vi "UIM Resolution.vi"() -> ()   [LabVIEW 2020]
doc: "This example shows how you could use UIM API to modify the resolution and layout of your application. Like this you can easily adapt your UI to different monitors."
uses:
  <vilib>/Utility/miscctls.llb/LVRectTypeDef.ctl
  UIM Class/UIM.lvclass
panel:
  in  "XML File":path caption="UIM XML Path"
  in  "Tab Control":enum32{"Page 1", "Page 2"}(tab)
  in  "Listbox":i32(listbox)
  in  "Play Button":bool
  in  "String":string
  out "Waveform Graph":dbl[](graph)
  in  "Stop Button":bool
  in  "UI State":u16(ring) items=["1024x768", "1600x900", "800x600"]
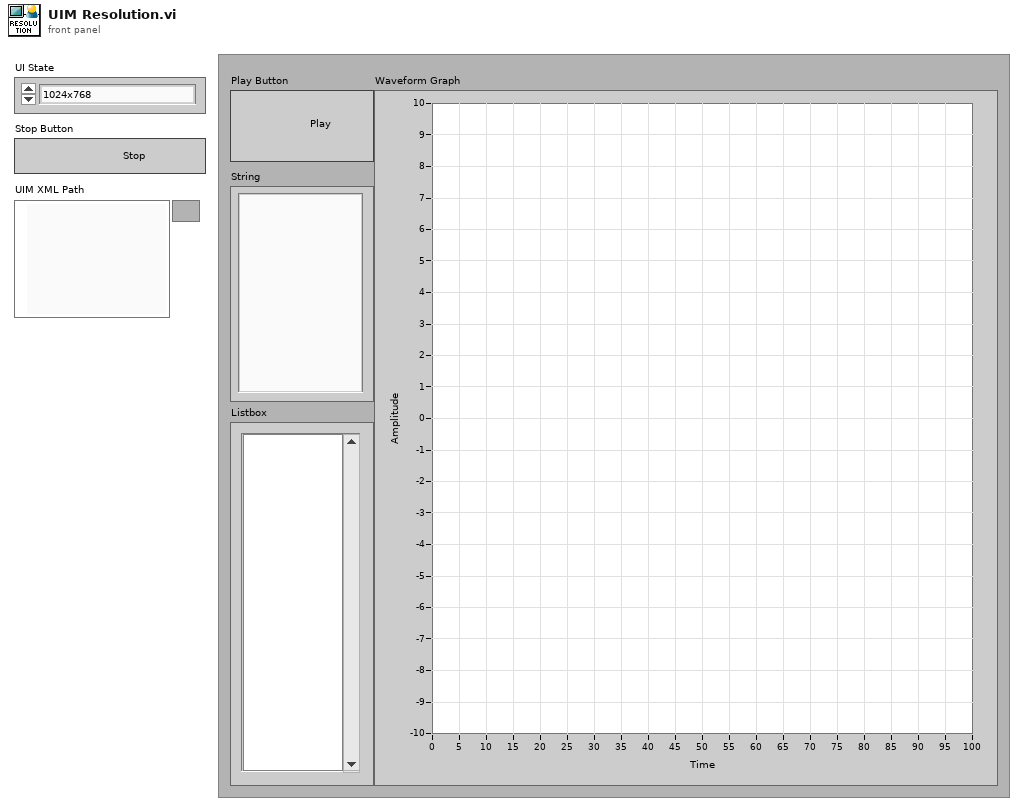
[diagram p1: front panel]
types:
  T1 = typedef "LVRectTypeDef.ctl" = cluster{"Left":i16, "Top":i16, "Right":i16, "Bottom":i16}
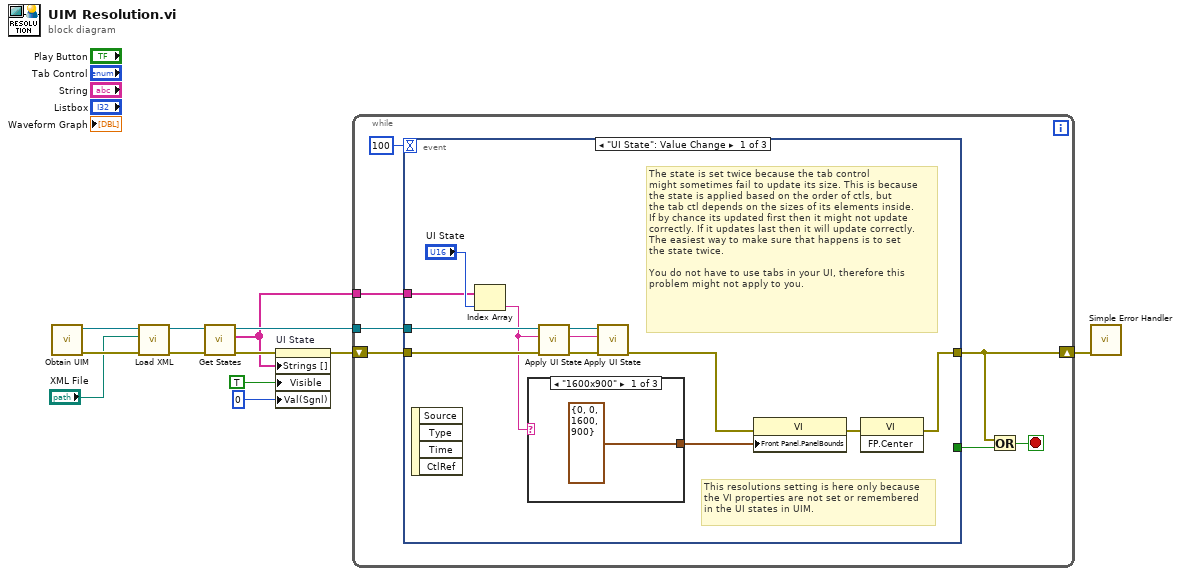
[diagram p0: block diagram]
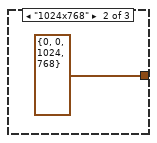
[diagram p2: hidden frame]
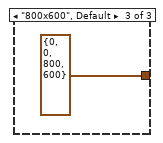
[diagram p3: hidden frame]
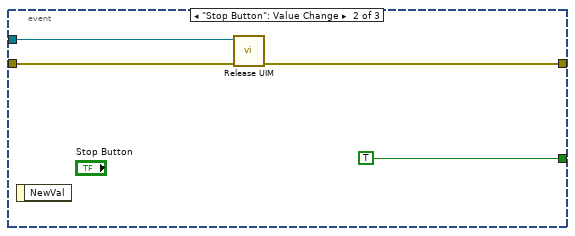
[diagram p4: hidden frame]
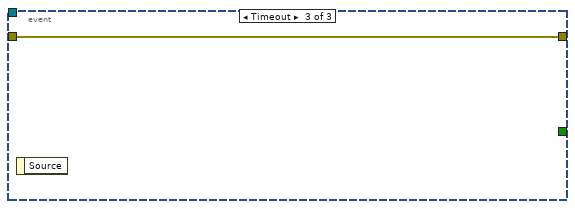
[diagram p5: hidden frame]
diagram:
  n1 = call "Obtain UIM.vi"() -> ("Error Out"=w3:errorcluster, "UIM Handle"=w8:refnum<data-value>)  [unwired: 10 in]
  n2 = call "Load XML.vi"("Error In"=w3, "XML File"="XML File", "UIM In"=w8) -> ("Error Out"=w4:errorcluster, "UIM Out"=w7:refnum<data-value>)  [unwired: 7 in]
  n3 = call "Get States.vi"("Error In"=w4, "UIM In"=w7) -> ("Error Out"=w5:errorcluster, "States"=w1:string[], "UIM Out"=w6:refnum<data-value>)  [unwired: 7 in]
  n4 = property on="UI State" class="Ring (strict)"(error in=w5, "Strings []"=w1, "Visible"=TRUE, "Val(Sgnl)"=u16 0 ("Value (Signaling)")) -> (error out=w12:errorcluster)  [unwired: 1 in, 1 out]
  n5 = while {
    tunnel: w6 -> [w19]
    tunnel: w1 -> [w17]
    shift-right: [w14] -> w9
    shift-left: w12 -> [w18]
    stop <- w15 stop-if-true
    n6 = event shown="[0] \"UI State\": Value Change" {
      selector: _ -> [_ _ _]
      dyn-events: _ -> [_ _ _]
      timeout: 100 -> [_ _ _]
      tunnel: w19 -> [w30 w36 _]
      tunnel: [_ TRUE _] -> w16
      tunnel: w18 -> [w29 w35 w38]
      tunnel: [w24 w34 w38] -> w14
      tunnel: w17 -> [w27 _ _]
      event "UI State": Value Change {
        # "The state is set twice because the tab control\nmight sometimes fail to update its size. This is because\nthe state is applied based on the order of ctls, but\nthe tab ctl depends on the sizes of its elements inside.\nIf by chance its updated first then it might not update\ncorrectly. If it updates last then it will update correctly.\nThe easiest way to make sure that happens is to set\nthe state twice.\n\nYou do not have to use tabs in your UI, therefore this\nproblem might not apply to you."
        # "This resolutions setting is here only because\nthe VI properties are not set or remembered\nin the UI states in UIM."
        n7 = event-data() -> ()  [unwired: 1 in, 4 out]
        n8 = Index Array(array=w27, index="UI State") -> (element=w20:string)
        n9 = case shown="\"1600x900\"" w20 {
          tunnel: [T1 {"Left"=0, "Top"=0, "Right"=1600, "Bottom"=900} ("Front Panel Window:Window Bounds") T1 {"Left"=0, "Top"=0, "Right"=1024, "Bottom"=768} ("Front Panel Window:Window Bounds") T1 {"Left"=0, "Top"=0, "Right"=800, "Bottom"=600} ("Front Panel Window:Window Bounds")] -> w26
          frame "1600x900" {
          }
          frame "1024x768" {
          }
          frame "800x600", Default {
          }
        }
        n10 = call "Apply UI State.vi"("Error In"=w29, "State Name"=w20, "UIM In"=w30) -> ("Error Out"=w23:errorcluster, "UIM Out"=w21:refnum<data-value>)  [unwired: 7 in]
        n11 = call "Apply UI State.vi"("Error In"=w23, "State Name"=w20, "UIM In"=w21) -> ("Error Out"=w22:errorcluster)  [unwired: 7 in, 1 out]
        n12 = property class="VI"(error in=w22, "Front Panel.PanelBounds"=w26) -> (error out=w25:errorcluster)  [unwired: 1 in, 1 out]
        n13 = invoke class="VI" method="FP.Center"(error in=w25) -> (error out=w24:errorcluster)  [unwired: 2 in, 2 out]
      }
      event "Stop Button": Value Change {
        n14 = event-data() -> ()  [unwired: 1 in, 1 out]
        n15 = call "Release UIM.vi"("Error In"=w35, "UIM Handle"=w36) -> ("Error Out"=w34:errorcluster)  [unwired: 9 in]
      }
      event Timeout {
        n16 = event-data() -> ()  [unwired: 1 in, 1 out]
      }
    }
    n17 = Or(x=w14, y=w16) -> (x .or. y?=w15:bool)
  }
  n18 = call <vilib>:"Simple Error Handler.vi"("error in (no error)"=w9) -> ()  [unwired: 4 in, 5 out]
